vi "zip_extract.vi"(6 "zip_extract_directory":path, 8 "error in (no error)":errorcluster, 11 "build_specifications":T1={"type"=enum."zip", "build_spec_name"="em-lv-NetworkStreams_Static", "target_name"="My Computer", "owner_name []"=[], "project_path"=path "D:/SourceControl/vi-packages/EM NetworkStreams/Source/NetworkStreams_Static/em-lv-NetworkStreams_Static.lvproj", "build_destination"=path "D:/SourceControl/vi-packages/EM NetworkStreams/Distribution/2014", "build_artifact"=path ""}) -> (0 "error out":errorcluster)   [LabVIEW 2015, in "lv-builder-default.lvlib"]
uses:
  lv-builder-default.lvlib
  lv-build/public/_controls/build_specification.ctl
  lv-build/public/_controls/build_type.ctl
  <userlib>/antonio-alexander/lv-bin-7zip/public/api/v1/advanced/extract_exe_archive.vi
  <userlib>/antonio-alexander/lv-bin/public/api/v1/v1.lvlib
  <userlib>/antonio-alexander/lv-bin-7zip/public/api/v1/v1.lvlib
  lv-build/lv-build.lvlib
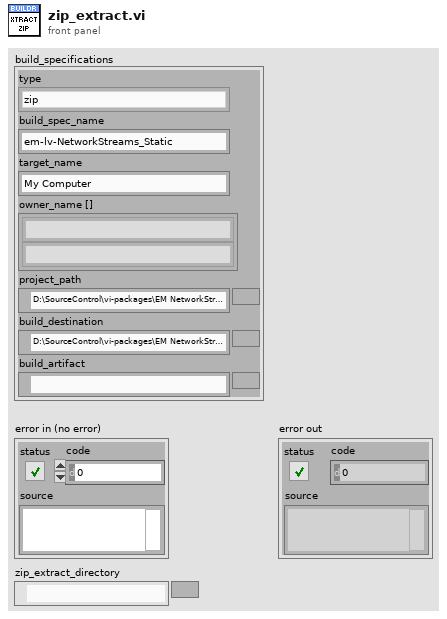
[diagram p1: front panel]
types:
  T1 = typedef "lv-build.lvlib/build_specification.ctl" = cluster{"type":T2, "build_spec_name":string, "target_name":string, "owner_name []":string[], "project_path":path, "build_destination":path, "build_artifact":path}
  T2 = typedef "lv-build.lvlib/build_type.ctl" = enum16{"<build_type>", "application_pc", "application_rt", "installer", "llb", "lvlibp", "zip", "fpga", "<null>"}
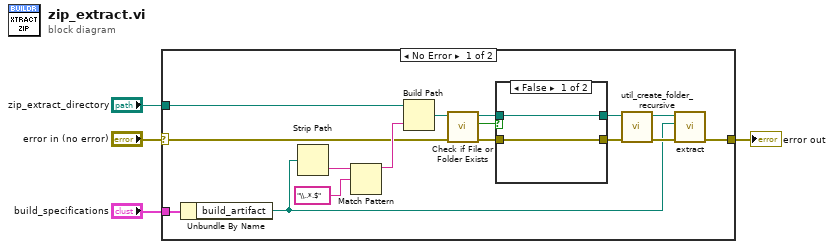
[diagram p0: block diagram]
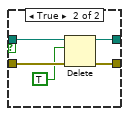
[diagram p2: hidden frame]
diagram:
  n1 = case shown="No Error" "error in (no error)" {
    selector: "error in (no error)" -> [w6 w28]
    tunnel: "build_specifications" -> [w19 _]
    tunnel: [w17 w28] -> w3
    tunnel: "zip_extract_directory" -> [w12 _]
    frame No Error {
      n2 = Unbundle By Name(w19) -> ("build_artifact"=w16:path)
      n3 = Strip Path(path=w16) -> (name=w15:string)  [unwired: 1 out]
      n4 = Match Pattern(string=w15, regular expression="\\..*.$") -> (before substring=w13:string)  [unwired: 1 in, 3 out]
      n5 = Build Path(base path=w12, name or relative path=w13) -> (appended path=w11:path)
      n6 = call <vilib>:"Check if File or Folder Exists.vi"("error in (no error)"=w6, "path"=w11) -> ("error out"=w9:errorcluster, "file or folder exists?"=w5:bool, "dup path"=w10:path)  [unwired: 7 in]
      n7 = case shown="False" w5 {
        tunnel: w10 -> [w22 w27]
        tunnel: w9 -> [w21 w26]
        tunnel: [w21 w25] -> w8
        tunnel: [w22 w24] -> w7
        frame False {
        }
        frame True {
          n8 = Delete(path (use dialog)=w27, entire hierarchy (F)=TRUE, error in=w26) -> (deleted path=w24:path, error out=w25:errorcluster)  [unwired: 2 in, 1 out]
        }
      }
      n9 = call <userlib>:"util_create_folder_recursive.vi"("error in"=w8, "path in"=w7) -> ("error out"=w20:errorcluster, "path out"=w18:path)  [unwired: 8 in]
      n10 = call-poly <userlib>:"extract.vi"("error in (no error)"=w20, "archive_path"=w16, "target_path in"=w18) -> ("error out"=w17:errorcluster)  [unwired: 5 in, 3 out]
    }
    frame Error {
    }
  }
  "error out" <- w3
